vi "Supported Type.vi"(9 "Error in":errorcluster caption="Error in (no error)", 11 "Variant":variant) -> (1 "Error out":errorcluster, 2 "Boolean":bool, 3 "Variant (dup)":variant)   [LabVIEW 2017, in "INI-Static-Variable-Support.lvlib"]
uses:
  INI-Static-Variable-Support.lvlib
  <vilib>/Utility/Data Type/NI_Data Type.lvlib
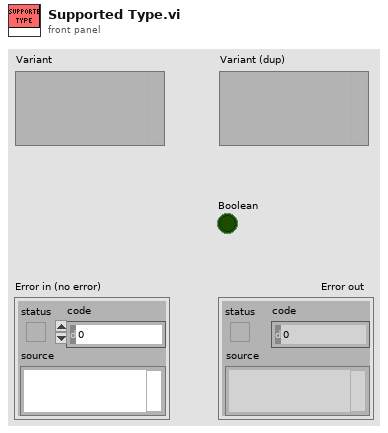
[diagram p1: front panel]
types:
  T1 = typedef "NI_Data Type.lvlib/Data Type.ctl" = enum8{"Invalid Type", "Void", "I8", "I16", "I32", "I64", "U8", "U16", "U32", "U64", "Single Float", "Double Float", "Extended Float", "Single Complex", "Double Complex", "Extended Complex", "Enum U8", "Enum U16", "Enum U32", "Enum U64", "Single Float With Unit", "Double Float With Unit", "Extended Float With Unit", "Single Complex with Unit", "Double Complex with Unit", "Extended Complex with Unit", "Boolean", "String", "Path", "Picture", "Tag", "Array", "Cluster", "Variant", "LV Variant", "Waveform", "Timestamp", "Digital Waveform", "Digital Data", "ExpressData", "Refnum", "External Data", "VI", "Poly VI", "LabVIEW Class Instance", "Fixed Point"}
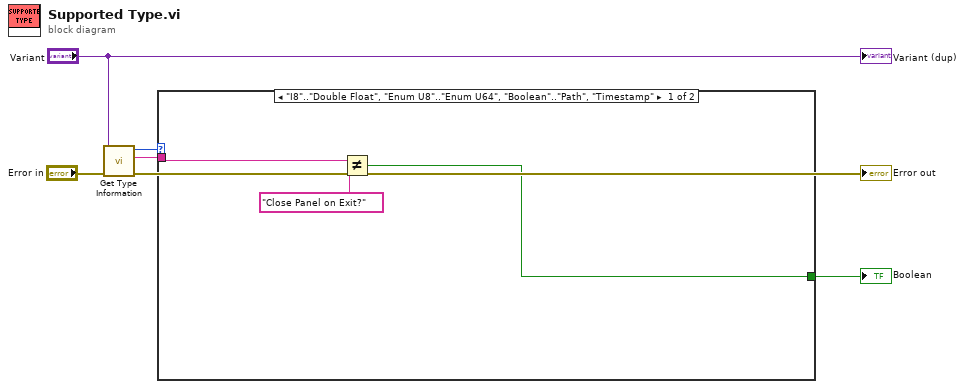
[diagram p0: block diagram]
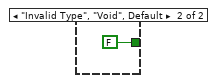
[diagram p2: hidden frame]
diagram:
  n1 = call <vilib>:"Get Type Information.vi"("error in (no error)"="Error in", "Variant"="Variant") -> ("error out"=→"Error out":errorcluster, "Name"=w4:string, "Type"=w5:T1)  [unwired: 5 in, 2 out]
  n2 = case shown="\"I8\"..\"Double Float\", \"Enum U8\"..\"Enum U64\", \"Boolean\"..\"Path\", \"Timestamp\"" w5 {
    tunnel: w4 -> [w9 _]
    tunnel: [w7 FALSE] -> w1
    frame "I8".."Double Float", "Enum U8".."Enum U64", "Boolean".."Path", "Timestamp" {
      n3 = Not Equal?(x=w9, y="Close Panel on Exit?") -> (x != y?=w7:bool)
    }
    frame "Invalid Type", "Void", Default {
    }
  }
  "Boolean" <- w1
  "Variant (dup)" <- "Variant"
